vi "Build Error Message.vi"(4 "Message Postfix":string, 6 "Error Messages":string[](array[string]), 11 "Error Code":i32) -> (3 "Error Message":string)   [LabVIEW 2016, in "Stream Error.lvlib" / "Error Interface.lvclass"]
doc: "--\nCopyright © 2017 Composed SystemsI All rights reserved.\n\nAuthor: Jon McBee <jon.mcbee@composed.io>\n\nThis library is provided \"AS IS\" ,WITHOUT WARRANTIES OR\nCONDITIONS OF ANY KIND, either express or implied.\n\nComposed Systems -- composed.io\n\nStream 0.0.1.1\nJon McBee - Composed Systems\nCopyright (c) 2017, Composed Systems"
uses:
  <userlib>/Composed Systems/Stream/Error/Classes/Error Interface/Error Interface.lvclass
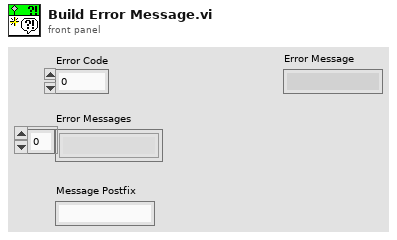
[diagram p1: front panel]
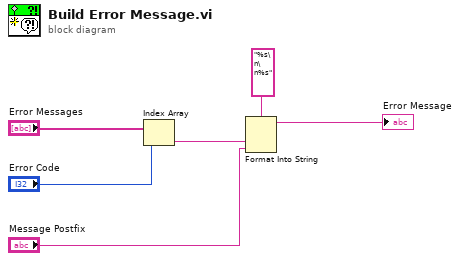
[diagram p0: block diagram]
diagram:
  n1 = Index Array(array="Error Messages", index="Error Code") -> (element=w3:string)
  n2 = Format Into String(format string="%s\n\n%s", w3, "Message Postfix") -> (resulting string=→"Error Message":string)  [unwired: 2 in, 1 out]
